vi "Recursive File List.vi"(4 "Folders to Exclude":string[](array[string]), 6 "pattern":string, 8 "error in (no error)":errorcluster, 9 "Continue Recursing on Error? (F)":bool, 10 "Treat LLBs as Folders?":bool, 11 "Folder Path":path) -> (0 "error out":errorcluster, 1 "Number of Files":i32, 2 "All Files in Dir":path[](array[path]), 3 "dup Folder Path":path, 5 "All Folders":path[](array[path]))   [LabVIEW 2019]
doc: "Lists the contents of a folder or LLB."
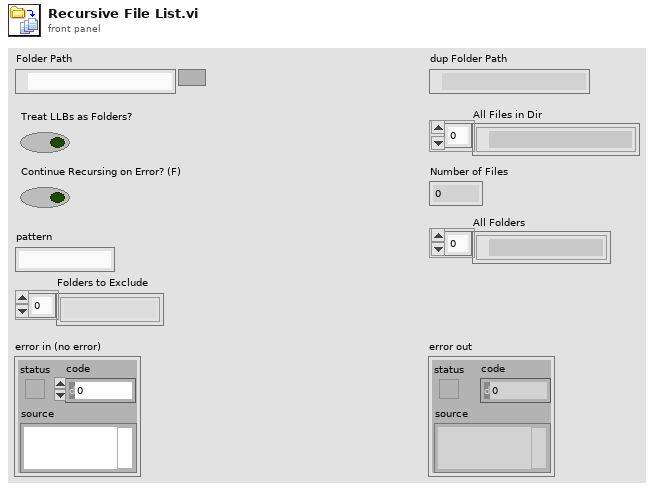
[diagram p1: front panel]
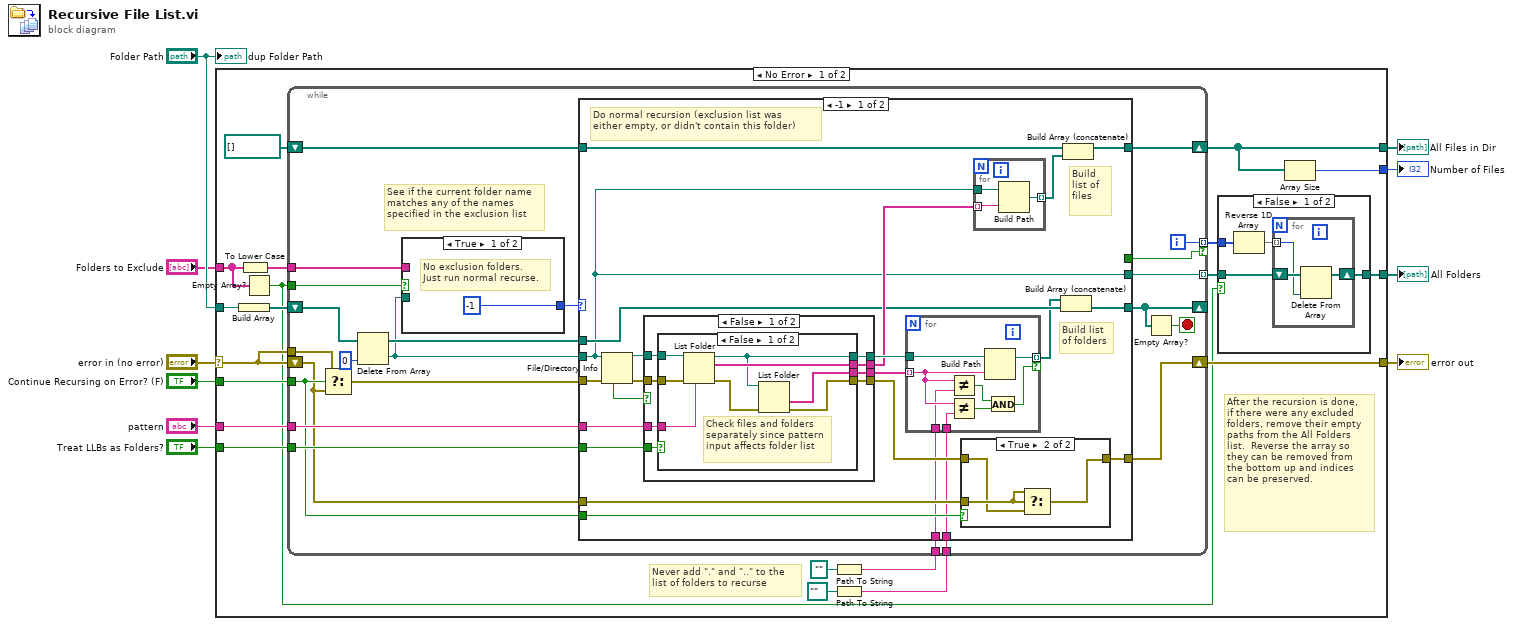
[diagram p0: block diagram]
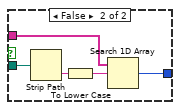
[diagram p2: hidden frame]
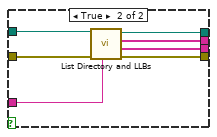
[diagram p3: hidden frame]
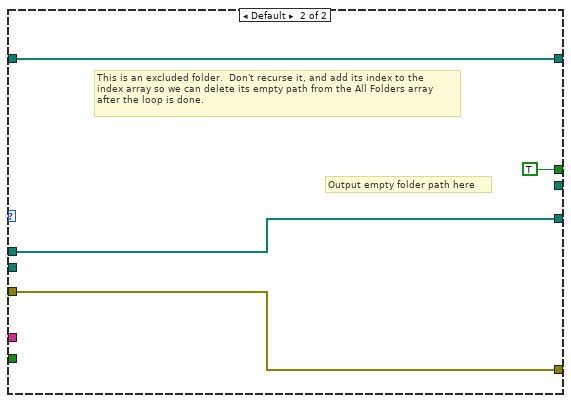
[diagram p6: hidden frame]
diagram:
  n1 = case shown="No Error" "error in (no error)" {
    selector: "error in (no error)" -> [w21 w134]
    tunnel: "Folder Path" -> [w30 _]
    tunnel: [w24 _] -> w10
    tunnel: [w23 _] -> w9
    tunnel: [w25 w134] -> w8
    tunnel: "Treat LLBs as Folders?" -> [w27 _]
    tunnel: [w18 _] -> w5
    tunnel: "pattern" -> [w26 _]
    tunnel: "Continue Recursing on Error? (F)" -> [w22 _]
    tunnel: "Folders to Exclude" -> [w16 _]
    frame No Error {
      # "Never add \".\" and \"..\" to the list of folders to recurse"
      # "After the recursion is done,\nif there were any excluded\nfolders, remove their empty\npaths from the All Folders\nlist.  Reverse the array so\nthey can be removed from\nthe bottom up and indices\ncan be preserved."
      n2 = Build Array(w30) -> (w29:path[])
      n3 = To Lower Case(string=w16) -> (all lower case string=w20:string[])
      n4 = Empty Array?(array=w16) -> (empty?=w15:bool)
      n5 = Path To String(path=path "") -> (string=w12:string)
      n6 = Path To String(path=path "..") -> (string=w11:string)
      n7 = while {
        shift-left: path[] [] ("Array Constant") -> [w51]
        shift-right: [w53] -> w24
        shift-left: w29 -> [w52]
        shift-right: [w48] -> _
        shift-right: [w42] -> w25
        shift-left: w21 -> [w41]
        tunnel: w27 -> [w50]
        tunnel: [w39] -> w19 mode=indexing
        tunnel: w26 -> [w49]
        tunnel: w22 -> [w43]
        tunnel: w21 -> [w44]
        tunnel: w20 -> [w37]
        tunnel: w15 -> [w38]
        tunnel: [w34] -> w17 mode=indexing if=w33
        tunnel: w12 -> [w32]
        tunnel: w11 -> [w31]
        i -> [w34]
        stop <- w47 stop-if-true
        # "See if the current folder name\nmatches any of the names\nspecified in the exclusion list"
        n8 = Select(t=w44, s=w43, f=w41) -> (s? t:f=w45:errorcluster)
        n9 = Delete From Array(array=w52, index=0) -> (deleted portion=w36:path, array with subset deleted=w40:path[])  [unwired: 1 in]
        n10 = case shown="True" w38 {
          tunnel: w37 -> [_ w56]
          tunnel: w36 -> [_ w59]
          tunnel: [-1 ("index of element") w55] -> w35
          frame True {
            # "No exclusion folders.\nJust run normal recurse."
          }
          frame False {
            n11 = Strip Path(path=w59) -> (name=w58:string)  [unwired: 1 out]
            n12 = To Lower Case(string=w58) -> (all lower case string=w57:string)
            n13 = Search 1D Array(1D array=w56, element=w57) -> (index of element=w55:i32)  [unwired: 1 out]
          }
        }
        n14 = case shown="-1" w35 {
          tunnel: [w81 w125] -> w53
          tunnel: w51 -> [w80 w125]
          tunnel: w50 -> [w78 _]
          tunnel: w49 -> [w77 _]
          tunnel: [w75 w124] -> w48
          tunnel: w36 -> [w64 _]
          tunnel: w45 -> [w71 w123]
          tunnel: w43 -> [w69 _]
          tunnel: [w68 w123] -> w42
          tunnel: w41 -> [w67 _]
          tunnel: w40 -> [w65 w124]
          tunnel: [w64 _] -> w39
          tunnel: [_ TRUE] -> w33
          tunnel: w32 -> [w61 _]
          tunnel: w31 -> [w60 _]
          frame -1 {
            # "Build list of files"
            # "Build list\nof folders"
            # "Do normal recursion (exclusion list was\neither empty, or didn't contain this folder)"
            n15 = File/Directory Info(path=w64, error in=w71) -> (path out=w73:path, error out=w74:errorcluster, shortcut=w72:bool)  [unwired: 4 out]
            n16 = case shown="False" w72 {
              tunnel: [w97 _] -> w66
              tunnel: [w96 w114] -> w79
              tunnel: [w95 w113] -> w70
              tunnel: w78 -> [w94 _]
              tunnel: w77 -> [w93 _]
              tunnel: [w92 _] -> w76
              tunnel: w74 -> [w91 w113]
              tunnel: w73 -> [w90 w114]
              frame False {
                n17 = case shown="False" w94 {
                  tunnel: [w105 w109] -> w97
                  tunnel: [w99 w108] -> w92
                  tunnel: w90 -> [w104 w112]
                  tunnel: [w98 w110] -> w96
                  tunnel: [w100 w107] -> w95
                  tunnel: w91 -> [w103 w111]
                  tunnel: w93 -> [w102 w106]
                  frame False {
                    # "Check files and folders\nseparately since pattern\ninput affects folder list"
                    n18 = List Folder(path=w104, pattern=w102, error in=w103) -> (path out=w98:path, filenames=w105:string[], error out=w101:errorcluster)  [unwired: 2 out]
                    n19 = List Folder(path=w98, error in=w101) -> (folder names=w99:string[], error out=w100:errorcluster)  [unwired: 4 out]
                  }
                  frame True {
                    n20 = call "List Directory and LLBs.vi"("pattern"=w106, "error in (no error)"=w111, "Folder Path"=w112) -> ("error out"=w107:errorcluster, "Folders and LLBs"=w108:string[], "Files sans LLBs"=w109:string[], "dup Folder Path"=w110:path)  [unwired: 5 out]
                  }
                }
              }
              frame True {
                # "Do not attempt to recurse the contents of folder shortcuts"
              }
            }
            n21 = for {
              tunnel: w79 -> [w89]
              tunnel: [w88] -> w63 mode=indexing if=w87
              tunnel: w76 -> [w86] mode=indexing
              tunnel: w61 -> [w85]
              tunnel: w60 -> [w84]
              n22 = Not Equal?(x=w86, y=w85) -> (x != y?=w82:bool)
              n23 = Not Equal?(x=w86, y=w84) -> (x != y?=w83:bool)
              n24 = Build Path(base path=w89, name or relative path=w86) -> (appended path=w88:path)
              n25 = And(x=w82, y=w83) -> (x .and. y?=w87:bool)
            }
            n26 = case shown="True" w69 {
              tunnel: w70 -> [w118 w120]
              tunnel: [w118 w119] -> w68
              tunnel: w67 -> [_ w121]
              frame False {
              }
              frame True {
                n27 = Select(t=w121, s=w121, f=w120) -> (s? t:f=w119:errorcluster)
              }
            }
            n28 = for {
              tunnel: w66 -> [w116] mode=indexing
              tunnel: w64 -> [w117]
              tunnel: [w115] -> w62 mode=indexing
              n29 = Build Path(base path=w117, name or relative path=w116) -> (appended path=w115:path)
            }
            n30 = Build Array (concatenate)(w63, w65) -> (w75:path[])
            n31 = Build Array (concatenate)(w80, w62) -> (w81:path[])
          }
          frame Default {
            # "Output empty folder path here"
            # "This is an excluded folder.  Don't recurse it, and add its index to the\nindex array so we can delete its empty path from the All Folders array\nafter the loop is done."
          }
        }
        n32 = Empty Array?(array=w48) -> (empty?=w47:bool)
      }
      n33 = case shown="False" w15 {
        tunnel: w19 -> [w128 w133]
        tunnel: [w127 w133] -> w18
        tunnel: w17 -> [w129 _]
        frame False {
          n34 = Reverse 1D Array(array=w129) -> (reversed array=w126:i32[])
          n35 = for {
            shift-right: [w131] -> w127
            shift-left: w128 -> [w132]
            tunnel: w126 -> [w130] mode=indexing
            n36 = Delete From Array(array=w132, index=w130) -> (array with subset deleted=w131:path[])  [unwired: 1 in, 1 out]
          }
        }
        frame True {
          # "No excluded folders.\nDon't run the code that\ndeletes excluded folder\nindices."
        }
      }
      n37 = Array Size(array=w24) -> (size(s)=w23:i32)
    }
    frame Error {
    }
  }
  "All Files in Dir" <- w10
  "Number of Files" <- w9
  "error out" <- w8
  "All Folders" <- w5
  "dup Folder Path" <- "Folder Path"
